vi "Teleop Cmd Send.vi"(0 "rt fifo":refnum<k33>, 1 "Teleop Inputs":T1, 2 "robolog":refnum<k34>, 3 "error in (no error)":errorcluster, 4 "Epsilon":dbl) -> (10 "error out":errorcluster)   [LabVIEW 2014]
uses:
  TeleopCmd.ctl
  CmdFlag.ctl
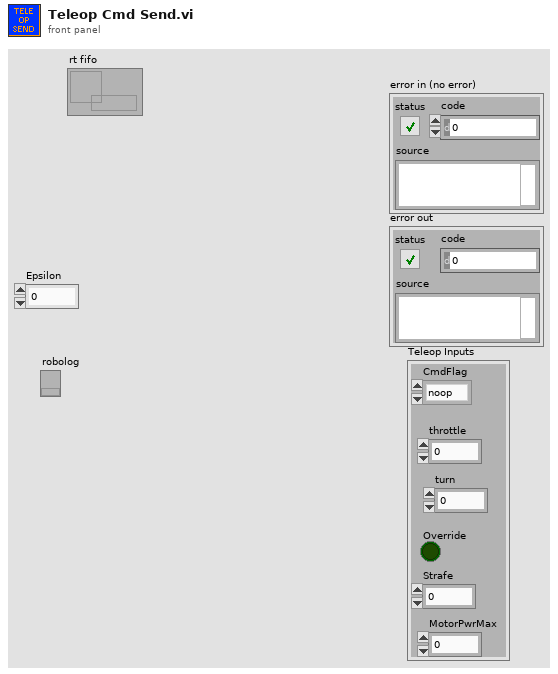
[diagram p1: front panel]
types:
  T1 = typedef "TeleopCmd.ctl" = cluster{"CmdFlag":T2, "throttle":dbl, "turn":dbl, "Override":bool, "Strafe":dbl, "MotorPwrMax":dbl}
  T2 = typedef "CmdFlag.ctl" = enum16{"noop", "suspend", "resume"}
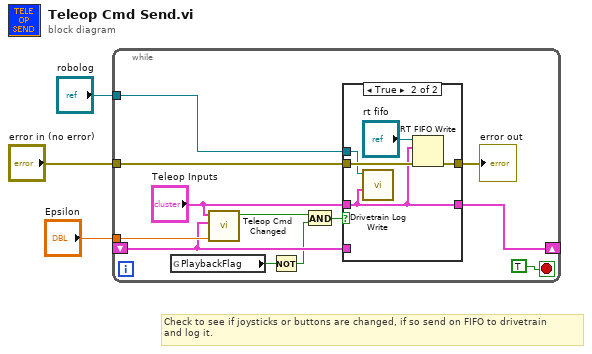
[diagram p0: block diagram]
diagram:
  # "Check to see if joysticks or buttons are changed, if so send on FIFO to drivetrain\nand log it."
  n1 = while "Prev Right\nPrev Right Value" {
    tunnel: "error in (no error)" -> [w14]
    tunnel: "Epsilon" -> [w12]
    shift-right: [w11] -> _
    shift-left: _ -> [w10]
    tunnel: "robolog" -> [w9]
    stop <- TRUE stop-if-true
    n2 = global read "PlaybackOn" "PlaybackFlag"() -> (w6:bool)
    n3 = call "Teleop Cmd Changed.vi"("Epsilon"=w12, "New Teleop Values"=w10, "Prev Teleop Values"="Teleop Inputs") -> ("Boolean"=w8:bool)  [unwired: 8 in]
    n4 = Not(x=w6) -> (.not. x?=w7:bool)
    n5 = And(x=w8, y=w7) -> (x .and. y?=w5:bool)
    n6 = case shown="True" w5 {
      tunnel: [w17 w22] -> w4
      tunnel: w14 -> [w17 w20]
      tunnel: "Teleop Inputs" -> [_ w18]
      tunnel: [w16 w18] -> w11
      tunnel: w10 -> [w16 _]
      tunnel: w9 -> [_ w19]
      frame False {
      }
      frame True {
        n7 = call "Drivetrain Log Write.vi"("Cluster"=w18, "robolog"=w19) -> ()  [unwired: 10 in]
        n8 = RT FIFO Write(0:"rt fifo", 1:w18, 3:w20) -> (11:w22:errorcluster)  [unwired: 2 in, 3 out]
      }
    }
    "error out" <- w4
  }
